vi "Periodic Tasks.vi"(8 "error in":errorcluster) -> ()   [LabVIEW 2015]
doc: "This VI runs in parallel to other robot code. It can contain as many user-defined periodic loops as you need. These can carry out PID or other sorts of timed response."
uses:
  <vilib>/Rock Robotics/WPI/Utilities/WPI_GetSetVariantRefNum.vi
  Drive/Implementation/Drive Published Globals.vi
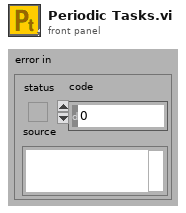
[diagram p1: front panel]
types:
  T1 = typedef "WPI_JoystickDevRef.ctl" = cluster{"Device":T2}
  T2 = typedef "WPI_JoystickDeviceEnum.ctl" = enum16{"USB 0", "USB 1", "USB 2", "USB 3", "USB 4", "USB 5"}
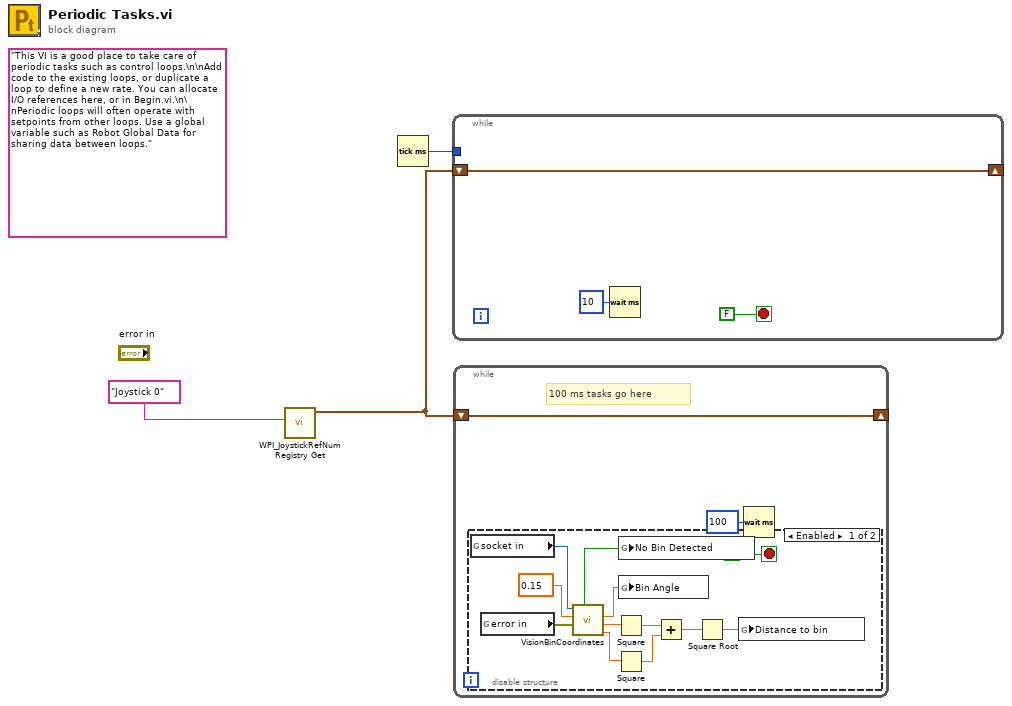
[diagram p0: block diagram]
diagram:
  (unwired) "This VI is a good place to take care of periodic tasks such as control loops.\n\nAdd code to the existing loops, or duplicate a loop to define a new rate. You can allocate I/O references here, or in Begin.vi.\n\nPeriodic loops will often operate with setpoints from other loops. Use a global variable such as Robot Global Data for sharing data between loops."
  n1 = call <vilib>:"WPI_JoystickRefNum Registry Get.vi"("refnum name"="Joystick 0") -> ("JoystickDevRef"=w2:T1)  [unwired: 1 in, 9 out]
  n2 = Tick Count (ms)() -> (millisecond timer value=w1:u32)
  n3 = while {
    shift-right: [w5] -> _
    shift-left: w2 -> [w5]
    tunnel: w1 -> [_]
    stop <- FALSE stop-if-true
    n4 = Wait (ms)(milliseconds to wait=u32 10) -> ()  [unwired: 1 out]
  }
  n5 = while {
    shift-right: [w7] -> _
    shift-left: w2 -> [w7]
    stop <- FALSE stop-if-true
    # "100 ms tasks go here"
    n6 = disable-structure shown="Enabled" {
      frame Enabled {
        n7 = global read "Drive Published Globals.vi" "socket in"() -> (w18:refnum<class "zmq_socket.lvclass">)
        n8 = global read "Drive Published Globals.vi" "error in"() -> (w19:errorcluster)
        n9 = call "VisionBinCoordinates.vi"("error in"=w19, "Minimum Ratio"=0.15, "socket in"=w18) -> ("x Coordinate of Bin"=w13:dbl, "y Coordinate of Bin"=w15:dbl, "bin angle"=w17:dbl, "no bin detected"=w16:bool)  [unwired: 1 in, 1 out]
        n10 = Square(x=w15) -> (x^2=w14:dbl)
        n11 = Square(x=w13) -> (x^2=w12:dbl)
        n12 = global write "Drive Published Globals.vi" "No Bin Detected"(w16) -> ()
        n13 = global write "Drive Published Globals.vi" "Bin Angle"(w17) -> ()
        n14 = Add(x=w14, y=w12) -> (x+y=w11:dbl)
        n15 = Square Root(x=w11) -> (sqrt(x)=w10:dbl)
        n16 = global write "Drive Published Globals.vi" "Distance to bin"(w10) -> ()
      }
      frame Disabled {
      }
    }
    n17 = Wait (ms)(milliseconds to wait=u32 100) -> ()  [unwired: 1 out]
  }
